vi "start Julia ZMQ server.vi"(8 "error in (no error)":errorcluster, 11 "Julia ZMQ server file name":string="ZMQ-testserver2.jl") -> (0 "error out":errorcluster, 3 "return code":i32)   [LabVIEW 2018, in "LV-Julia_ZMQ-Roundtrip_lib.lvlib"]
uses:
  LV-Julia_ZMQ-Roundtrip_lib.lvlib
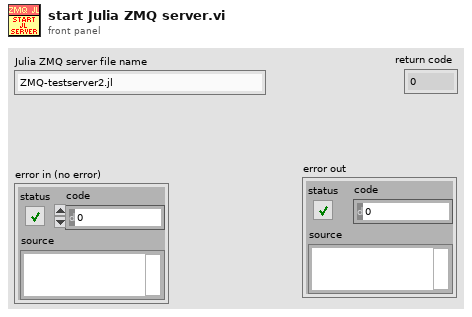
[diagram p1: front panel]
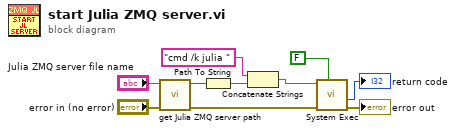
[diagram p0: block diagram]
diagram:
  n1 = call "get Julia ZMQ server path.vi"("error in (no error)"="error in (no error)", "Julia ZMQ server file name"="Julia ZMQ server file name") -> ("error out"=w8:errorcluster, "Julia ZMQ server file path"=w5:path)  [unwired: 8 in]
  n2 = Path To String(path=w5) -> (string=w3:string)
  n3 = Concatenate Strings("cmd /k julia ", w3) -> (w2:string)
  n4 = call <vilib>:"System Exec.vi"("wait until completion? (T)"=FALSE, "error in (no error)"=w8, "command line"=w2) -> ("error out"=→"error out":errorcluster, "return code"=→"return code":i32)  [unwired: 5 in, 2 out]
